vi "Write IoU.vi"(8 "error in (no error)":errorcluster, 10 "IoU":sgl, 11 "ONNX YOLO Class in":refnum<class "ONNX YOLO Class.lvclass">) -> (0 "error out":errorcluster, 3 "ONNX YOLO Class out":refnum<class "ONNX YOLO Class.lvclass">)   [LabVIEW 2017, in "ONNX YOLO Class Library.lvlib" / "ONNX YOLO Class.lvclass"]
uses:
  ONNX YOLO Class.lvclass
  ONNX YOLO Class.lvclass/ONNX YOLO Class.ctl
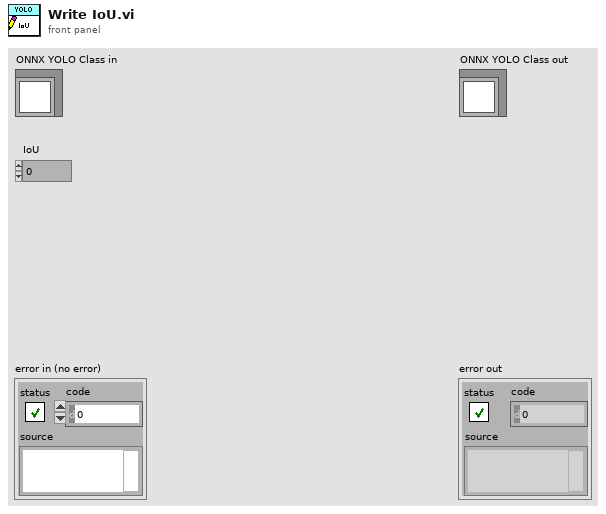
[diagram p1: front panel]
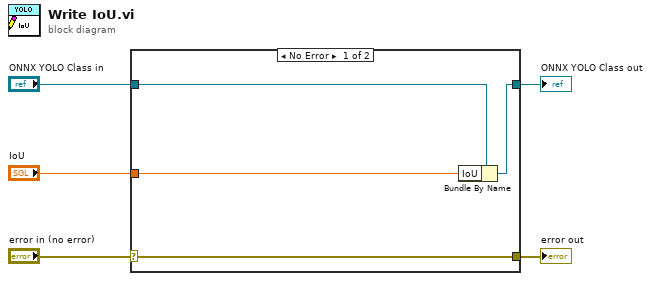
[diagram p0: block diagram]
diagram:
  n1 = case shown="No Error" "error in (no error)" {
    selector: "error in (no error)" -> [w9 w10]
    tunnel: [w9 w10] -> w4
    tunnel: [w7 w11] -> w2
    tunnel: "ONNX YOLO Class in" -> [w8 w11]
    tunnel: "IoU" -> [w6 _]
    frame No Error {
      n2 = Bundle By Name(cluster=w8, "IoU"=w6) -> (w7:refnum<class "ONNX YOLO Class.lvclass">)
    }
    frame Error {
    }
  }
  "error out" <- w4
  "ONNX YOLO Class out" <- w2
